vi "ex01.vi"() -> ()   [LabVIEW 2011]
panel:
  out "Array":void[](array[numeric])
  in  "loops":dbl
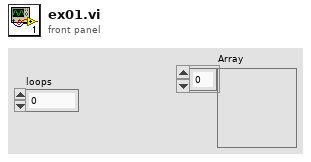
[diagram p1: front panel]
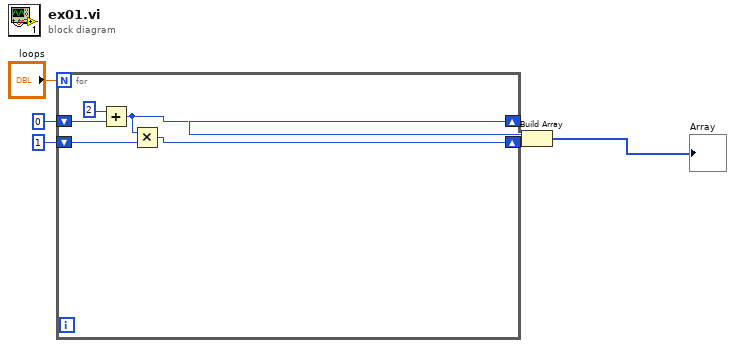
[diagram p0: block diagram]
diagram:
  n1 = for {
    N: "loops" -> [_]
    shift-right: [w8] -> w3
    shift-left: 0 -> [w10]
    shift-right: [w7] -> w2
    shift-left: 1 -> [w9]
    n2 = Add(x=2, y=w10) -> (x+y=w8:i32)
    n3 = Multiply(x=w8, y=w9) -> (x*y=w7:i32)
  }
  n4 = Build Array(w3, w2) -> (→"Array":i32[])
